vi "FallTimeInterval.vi"(11 "Fall Time Interval":dbl format="%.6f") -> (3 "Time interval in Hex":u32 format="%x")   [LabVIEW 2016]
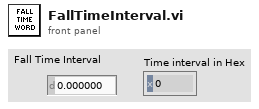
[diagram p1: front panel]
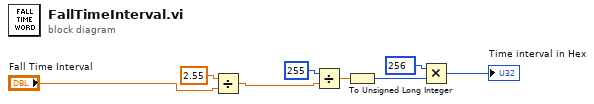
[diagram p0: block diagram]
diagram:
  n1 = Divide(x=2.55, y="Fall Time Interval") -> (x/y=w3:dbl)
  n2 = Divide(x=u32 255, y=w3) -> (x/y=w8:dbl)
  n3 = To Unsigned Long Integer(number=w8) -> (unsigned 32bit integer=w5:u32)
  n4 = Multiply(x=u32 256, y=w5) -> (x*y=→"Time interval in Hex":u32)
